vi "Copy and Modify Template Plugin.vi"(8 "error in":errorcluster, 10 "template library path":path, 11 "configuration":T1) -> (0 "error out":errorcluster)   [LabVIEW 2021, in "InstrumentStudio Plug-In Editor.lvlib"]
uses:
  InstrumentStudio Plug-In Editor.lvlib
  Data Holder.ctl
  Error Strings Global Internal.vi
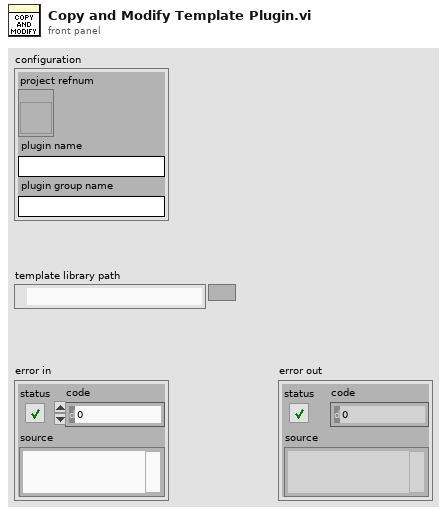
[diagram p1: front panel]
types:
  T1 = typedef "InstrumentStudio Plug-In Editor.lvlib/Data Holder.ctl" = cluster{"project refnum":refnum<vi>, "plugin name":string, "plugin group name":string}
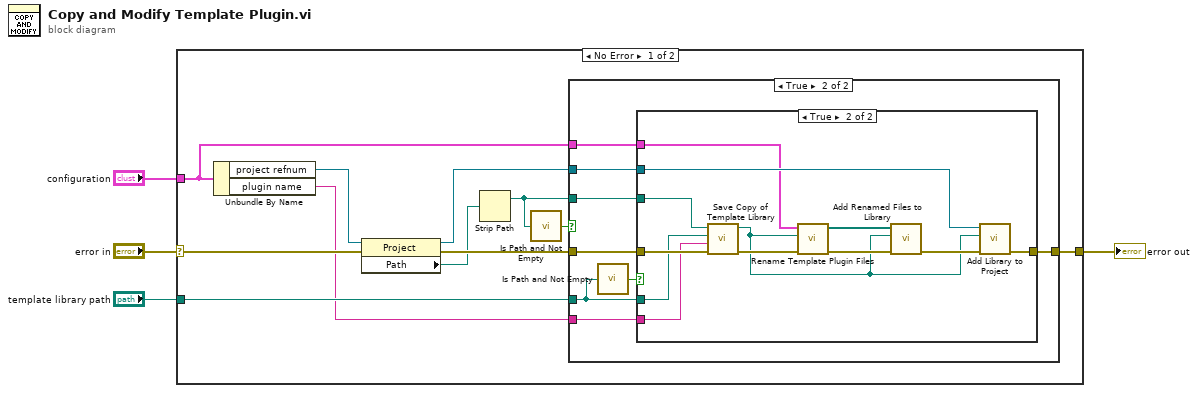
[diagram p0: block diagram]
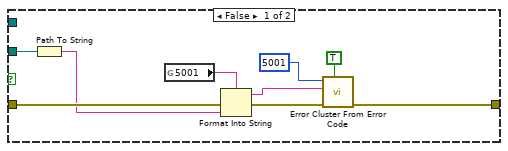
[diagram p2: hidden frame]
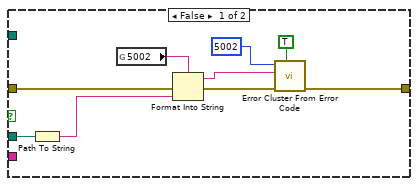
[diagram p3: hidden frame]
diagram:
  n1 = case shown="No Error" "error in" {
    selector: "error in" -> [w11 w54]
    tunnel: "template library path" -> [w15 _]
    tunnel: "configuration" -> [w13 _]
    tunnel: [w6 w54] -> w2
    frame No Error {
      n2 = Unbundle By Name(w13) -> ("project refnum"=w14:refnum<vi>, "plugin name"=w7:string)
      n3 = property class="Project"(reference=w14, error in=w11) -> (reference out=w12:refnum<vi>, error out=w10:errorcluster, "Path"=w9:path)
      n4 = Strip Path(path=w9) -> (stripped path=w5:path)  [unwired: 1 out]
      n5 = call <vilib>:"Is Path and Not Empty.vi"("path"=w5) -> ("Is Path and Not Empty?"=w8:bool)  [unwired: 4 in]
      n6 = case shown="True" w8 {
        tunnel: w15 -> [_ w25]
        tunnel: w5 -> [w16 w32]
        tunnel: w13 -> [_ w31]
        tunnel: w12 -> [_ w30]
        tunnel: w10 -> [w18 w29]
        tunnel: [w19 w28] -> w6
        tunnel: w7 -> [_ w26]
        frame False {
          n7 = Path To String(path=w16) -> (string=w17:string)
          n8 = global read "Error Strings Global Internal.vi" "5001"() -> (w22:string)
          n9 = Format Into String(format string=w22, error in=w18, w17) -> (resulting string=w23:string, error out=w24:errorcluster)  [unwired: 1 in]
          n10 = call <vilib>:"Error Cluster From Error Code.vi"("show call chain? (False)"=TRUE, "error in (no error)"=w24, "error message (\"\")"=w23, "error code (0)"=5001) -> ("error out"=w19:errorcluster)  [unwired: 5 in]
        }
        frame True {
          n11 = call <vilib>:"Is Path and Not Empty.vi"("path"=w25) -> ("Is Path and Not Empty?"=w27:bool)  [unwired: 4 in]
          n12 = case shown="True" w27 {
            tunnel: w32 -> [_ w48]
            tunnel: w31 -> [_ w42]
            tunnel: w30 -> [_ w44]
            tunnel: w29 -> [w40 w53]
            tunnel: [w39 w49] -> w28
            tunnel: w25 -> [w33 w47]
            tunnel: w26 -> [_ w46]
            frame False {
              n13 = Path To String(path=w33) -> (string=w34:string)
              n14 = global read "Error Strings Global Internal.vi" "5002"() -> (w37:string)
              n15 = Format Into String(format string=w37, error in=w40, w34) -> (resulting string=w38:string, error out=w41:errorcluster)  [unwired: 1 in]
              n16 = call <vilib>:"Error Cluster From Error Code.vi"("show call chain? (False)"=TRUE, "error in (no error)"=w41, "error message (\"\")"=w38, "error code (0)"=5002) -> ("error out"=w39:errorcluster)  [unwired: 5 in]
            }
            frame True {
              n17 = call "Save Copy of Template Library.vi"("error in"=w53, "plugin name"=w46, "template library path"=w47, "project path"=w48) -> ("error out"=w52:errorcluster, "plugin library path"=w45:path)  [unwired: 6 in]
              n18 = call "Rename Template Plugin Files.vi"("error in"=w52, "plugin library path"=w45, "configuration"=w42) -> ("error out"=w51:errorcluster, "plugin files path"=w43:path[])  [unwired: 7 in]
              n19 = call "Add Renamed Files to Library.vi"("error in"=w51, "plugin library path"=w45, "plugin files path"=w43) -> ("error out"=w50:errorcluster)  [unwired: 8 in]
              n20 = call "Add Library to Project.vi"("error in"=w50, "plugin library path"=w45, "project refnum"=w44) -> ("error out"=w49:errorcluster)  [unwired: 8 in]
            }
          }
        }
      }
    }
    frame Error {
    }
  }
  "error out" <- w2
